vi "encodeInt32.vi"(2 "Compress? (T)":bool=TRUE, 3 "Int32":i32) -> (1 "MessagePack":u8[](array[numeric]) format="%.0x")   [LabVIEW 2015, in "MsgPack.lvlib"]
uses:
  MsgPack.lvlib
  encodeInt8.vi
  SubVis/encodeFixedInt.vi
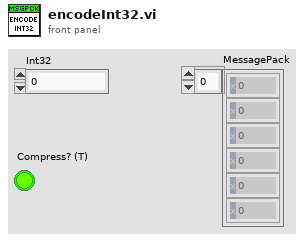
[diagram p1: front panel]
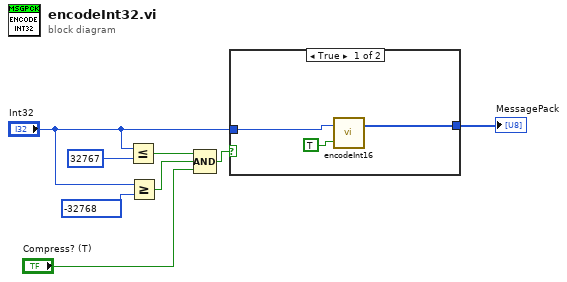
[diagram p0: block diagram]
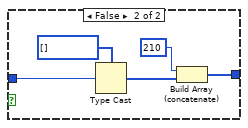
[diagram p2: hidden frame]
diagram:
  n1 = Less Or Equal?(x="Int32", y=32767) -> (x <= y?=w5:bool)
  n2 = Greater Or Equal?(x="Int32", y=-32768) -> (x >= y?=w4:bool)
  n3 = Compound Arithmetic op=AND(w5, w4, "Compress? (T)") -> (w2:bool)
  n4 = case shown="True" w2 {
    tunnel: [w10 w16] -> w8
    tunnel: "Int32" -> [w11 w12]
    frame True {
      n5 = call "encodeInt16.vi"("Compress? (T)"=TRUE ("Compress"), "Int16"=w11) -> ("MessagePack"=w10:u8[])  [unwired: 1 in]
    }
    frame False {
      n6 = Type Cast(type=u8[] [], x=w12) -> (*(type *) &x=w13:u8[])
      n7 = Build Array (concatenate)(u8 210, w13) -> (w16:u8[])
    }
  }
  "MessagePack" <- w8
